vi "PXI-Prepare AO Gains OTF.vi"(8 "error in (no error)":errorcluster, 11 "Gains":dbl[](array[numeric])) -> (0 "error out":errorcluster)   [LabVIEW 2015]
uses:
  PXI Globals.vi
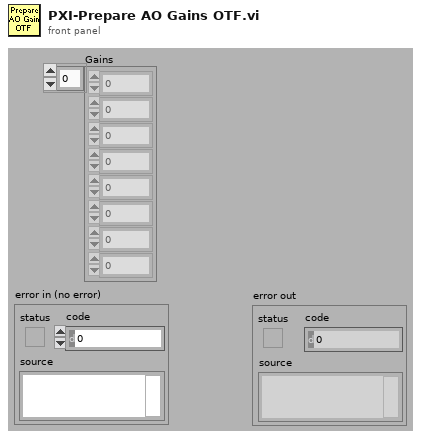
[diagram p1: front panel]
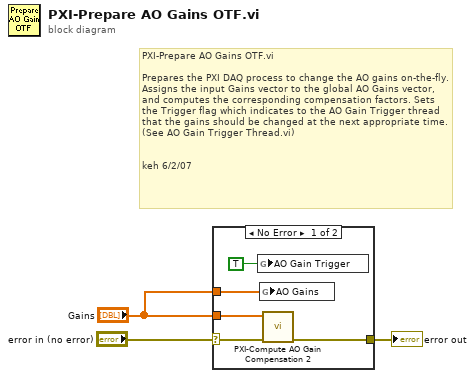
[diagram p0: block diagram]
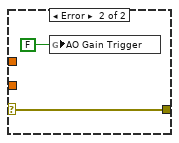
[diagram p2: hidden frame]
diagram:
  # "PXI-Prepare AO Gains OTF.vi\n\nPrepares the PXI DAQ process to change the AO gains on-the-fly. Assigns the input Gains vector to the global AO Gains vector, and computes the corresponding compensation factors. Sets the Trigger flag which indicates to the AO Gain Trigger thread that the gains should be changed at the next appropriate time. (See AO Gain Trigger Thread.vi)\n\n\nkeh 6/2/07"
  n1 = case shown="No Error" "error in (no error)" {
    selector: "error in (no error)" -> [w8 w10]
    tunnel: [w7 w10] -> w2
    tunnel: "Gains" -> [w6 _]
    tunnel: "Gains" -> [w4 _]
    frame No Error {
      n2 = global write "PXI Globals.vi" "AO Gain Trigger"(TRUE) -> ()
      n3 = global write "PXI Globals.vi" "AO Gains"(w4) -> ()
      n4 = call "PXI-Compute AO Gain Compensation 2.vi"("error in (no error)"=w8, "Gains"=w6) -> ("error out"=w7:errorcluster)  [unwired: 9 in]
    }
    frame Error {
      n5 = global write "PXI Globals.vi" "AO Gain Trigger"(FALSE) -> ()
    }
  }
  "error out" <- w2
